vi "CRYSearch for Intersection.vi"(4 "All points":bool, 6 "Search range":string[](array[string]), 7 "Supress warnings (F)":bool, 9 "Operand B":T1={"Name"="", "Curve"=[], "X data"=1, "Y data"=1, "Z data"=1, "X axis"=0, "Y axis"=1, "Z axis"=1, "X unit"="Hz", "Y unit"="", "Z unit"="deg.", "X dB ref"=1.0, "Y dB ref"=1.0, "Z dB ref"=1.0, "single val"=FALSE, "protected"=FALSE, "display X"=TRUE, "display Y"=TRUE, "display Z"=TRUE, "Test Info"="", "Step No."=0, "Plot Settings"={"Color"=0, "Interpolation"=0, "Point Style"=0, "Line Style"=0, "Point Color"=0, "Line Width"=0, "Bar Plot Style"=0, "Fill To"=0}, "AutoProtect"=FALSE} {"Z data" items=["dB", "Lin"]; "X data" items=["dB", "Lin"]; "Y data" items=["dB", "Lin"]; "Z dB ref" format="%.1f"; "Z axis" items=["Log", "Lin"]; "X dB ref" format="%.1f"; "X axis" items=["Log", "Lin"]; "Y axis" items=["Log", "Lin"]; "Y dB ref" format="%.1f"; "Curve"."z" format="%.2f"; "Curve"."y" format="%.2f"; "Curve"."x" format="%.2f"}, 11 "Operand A":T1={"Name"="", "Curve"=[], "X data"=1, "Y data"=1, "Z data"=1, "X axis"=0, "Y axis"=1, "Z axis"=1, "X unit"="Hz", "Y unit"="", "Z unit"="deg.", "X dB ref"=1.0, "Y dB ref"=1.0, "Z dB ref"=1.0, "single val"=FALSE, "protected"=FALSE, "display X"=TRUE, "display Y"=TRUE, "display Z"=TRUE, "Test Info"="", "Step No."=0, "Plot Settings"={"Color"=0, "Interpolation"=0, "Point Style"=0, "Line Style"=0, "Point Color"=0, "Line Width"=0, "Bar Plot Style"=0, "Fill To"=0}, "AutoProtect"=FALSE} {"Z data" items=["dB", "Lin"]; "X data" items=["dB", "Lin"]; "Y data" items=["dB", "Lin"]; "Z dB ref" format="%.1f"; "Z axis" items=["Log", "Lin"]; "X dB ref" format="%.1f"; "X axis" items=["Log", "Lin"]; "Y axis" items=["Log", "Lin"]; "Y dB ref" format="%.1f"; "Curve"."z" format="%.2f"; "Curve"."y" format="%.2f"; "Curve"."x" format="%.2f"}) -> (3 "Resulting data":T1={"Name"="", "Curve"=[], "X data"=1, "Y data"=1, "Z data"=1, "X axis"=0, "Y axis"=1, "Z axis"=1, "X unit"="Hz", "Y unit"="", "Z unit"="deg.", "X dB ref"=1.0, "Y dB ref"=1.0, "Z dB ref"=1.0, "single val"=FALSE, "protected"=FALSE, "display X"=TRUE, "display Y"=TRUE, "display Z"=TRUE, "Test Info"="", "Step No."=0, "Plot Settings"={"Color"=0, "Interpolation"=0, "Point Style"=0, "Line Style"=0, "Point Color"=0, "Line Width"=0, "Bar Plot Style"=0, "Fill To"=0}, "AutoProtect"=FALSE} {"Z data" items=["dB", "Lin"]; "X data" items=["dB", "Lin"]; "Y data" items=["dB", "Lin"]; "Z dB ref" format="%.1f"; "Z axis" items=["Log", "Lin"]; "X dB ref" format="%.1f"; "X axis" items=["Log", "Lin"]; "Y axis" items=["Log", "Lin"]; "Y dB ref" format="%.1f"; "Curve"."z" format="%.2f"; "Curve"."y" format="%.2f"; "Curve"."x" format="%.2f"})   [LabVIEW 2013]
uses:
  Typedef Control/CRYData Cluster.ctl
  <vilib>/Analysis/7linalg.llb/Solve Linear Equations (single right hand).vi
  <vilib>/Analysis/baseanly.llb/Solve Linear Equations By Cholesky.vi
  <vilib>/Analysis/baseanly.llb/Real Matrix to Compact Array.vi
  <vilib>/Analysis/baseanly.llb/Real Compact Tri-Matrix Linear Eqs.vi
  <vilib>/Analysis/7linalg.llb/Solve Linear Eqs (General).vi
  <vilib>/Analysis/7linalg.llb/Solve Linear Eqs (Gen, single right hand).vi
  <vilib>/Analysis/NI_AALPro.lvlib
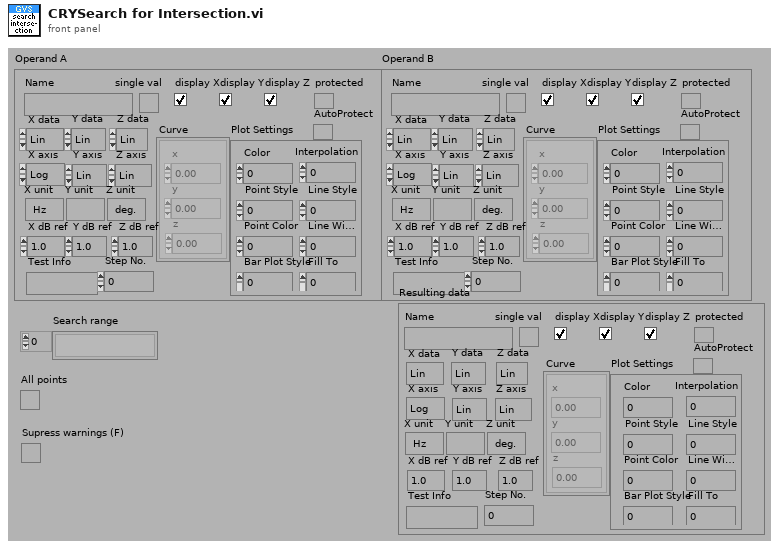
[diagram p1: front panel]
types:
  T1 = typedef "CRYData Cluster.ctl" = cluster{"Name":string, "Curve":cluster{"x":dbl, "y":dbl, "z":dbl}[], "X data":u16, "Y data":u16, "Z data":u16, "X axis":u16, "Y axis":u16, "Z axis":u16, "X unit":string, "Y unit":string, "Z unit":string, "X dB ref":dbl, "Y dB ref":dbl, "Z dB ref":dbl, "single val":bool, "protected":bool, "display X":bool, "display Y":bool, "display Z":bool, "Test Info":string, "Step No.":i32, "Plot Settings":cluster{"Color":u32, "Interpolation":u8, "Point Style":u8, "Line Style":u8, "Point Color":u32, "Line Width":u8, "Bar Plot Style":u8, "Fill To":i16}, "AutoProtect":bool}
  T2 = enum16{"OK", "Yes", "YesNo", "YesNoCancel", "ReplaceAppend"}
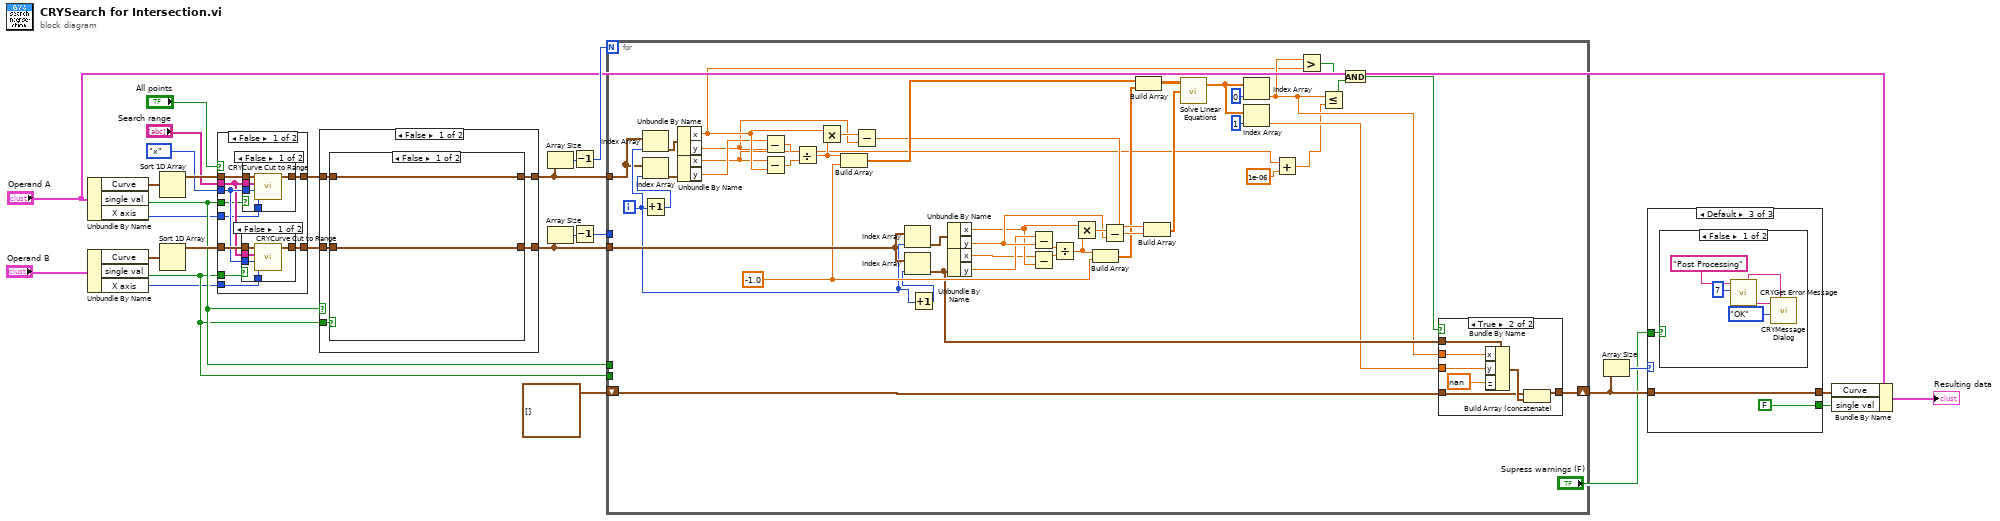
[diagram p0: block diagram]
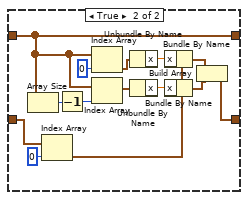
[diagram p2: hidden frame]
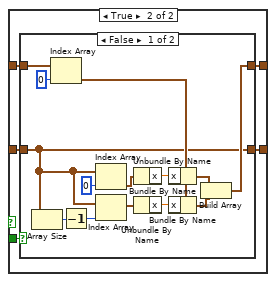
[diagram p3: hidden frame]
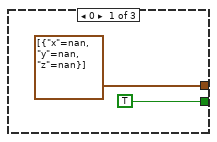
[diagram p5: hidden frame]
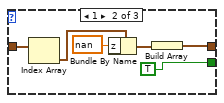
[diagram p6: hidden frame]
diagram:
  n1 = Unbundle By Name("Operand A") -> ("Curve"=w28:cluster{"x":dbl, "y":dbl, "z":dbl}[], "single val"=w9:bool, "X axis"=w7:u16)
  n2 = Unbundle By Name("Operand B") -> ("Curve"=w23:cluster{"x":dbl, "y":dbl, "z":dbl}[], "single val"=w8:bool, "X axis"=w6:u16)
  n3 = Sort 1D Array(array=w28) -> (sorted array=w27:cluster{"x":dbl, "y":dbl, "z":dbl}[])
  n4 = Sort 1D Array(array=w23) -> (sorted array=w22:cluster{"x":dbl, "y":dbl, "z":dbl}[])
  n5 = case shown="False" "All points" {
    tunnel: w27 -> [w38 w52]
    tunnel: [w37 w52] -> w13
    tunnel: enum16{"x", "y", "z"}."x" ("Range variable") -> [w35 _]
    tunnel: "Search range" -> [w34 _]
    tunnel: w22 -> [w36 w51]
    tunnel: [w33 w51] -> w11
    tunnel: w9 -> [w32 _]
    tunnel: w8 -> [w31 _]
    tunnel: w7 -> [w30 _]
    tunnel: w6 -> [w29 _]
    frame False {
      n6 = case shown="False" w31 {
        tunnel: w36 -> [w43 w44]
        tunnel: w35 -> [w42 _]
        tunnel: w34 -> [w41 _]
        tunnel: [w40 w44] -> w33
        tunnel: w29 -> [w39 _]
        frame False {
          n7 = call "CRYCurve Cut to Range.vi"("Axis type (Lin)"=w39, "Range variable (x)"=w42, "Search range"=w41, "Curve in"=w43) -> ("Cut curve out"=w40:cluster{"x":dbl, "y":dbl, "z":dbl}[])  [unwired: 7 out]
        }
        frame True {
        }
      }
      n8 = case shown="False" w32 {
        tunnel: w38 -> [w49 w50]
        tunnel: [w48 w50] -> w37
        tunnel: w35 -> [w47 _]
        tunnel: w34 -> [w46 _]
        tunnel: w30 -> [w45 _]
        frame False {
          n9 = call "CRYCurve Cut to Range.vi"("Axis type (Lin)"=w45, "Range variable (x)"=w47, "Search range"=w46, "Curve in"=w49) -> ("Cut curve out"=w48:cluster{"x":dbl, "y":dbl, "z":dbl}[])  [unwired: 7 out]
        }
        frame True {
        }
      }
    }
    frame True {
    }
  }
  n10 = case shown="False" w9 {
    tunnel: w8 -> [w57 w78]
    tunnel: w13 -> [w56 w77]
    tunnel: [w55 w76] -> w12
    tunnel: w11 -> [w54 w75]
    tunnel: [w53 w74] -> w10
    frame False {
      n11 = case shown="False" w57 {
        tunnel: [w59 w61] -> w55
        tunnel: w56 -> [w59 w61]
        tunnel: [w58 w60] -> w53
        tunnel: w54 -> [w58 w63]
        frame False {
        }
        frame True {
          n12 = Array Size(array=w61) -> (size(s)=w73:i32)
          n13 = Index Array(array=w63, index=0 ("Index")) -> (element=w62:cluster{"x":dbl, "y":dbl, "z":dbl})
          n14 = Decrement(x=w73) -> (x-1=w71:i32)
          n15 = Index Array(array=w61, index=0 ("Index")) -> (element=w69:cluster{"x":dbl, "y":dbl, "z":dbl})
          n16 = Index Array(array=w61, index=w71) -> (element=w68:cluster{"x":dbl, "y":dbl, "z":dbl})
          n17 = Unbundle By Name(w69) -> ("x"=w67:dbl)
          n18 = Unbundle By Name(w68) -> ("x"=w66:dbl)
          n19 = Bundle By Name(cluster=w62, "x"=w67) -> (w65:cluster{"x":dbl, "y":dbl, "z":dbl})
          n20 = Bundle By Name(cluster=w62, "x"=w66) -> (w64:cluster{"x":dbl, "y":dbl, "z":dbl})
          n21 = Build Array(w65, w64) -> (w60:cluster{"x":dbl, "y":dbl, "z":dbl}[])
        }
      }
    }
    frame True {
      n22 = case shown="False" w78 {
        tunnel: [w80 w94] -> w76
        tunnel: w77 -> [w88 w94]
        tunnel: [w79 w93] -> w74
        tunnel: w75 -> [w79 w93]
        frame False {
          n23 = Array Size(array=w79) -> (size(s)=w92:i32)
          n24 = Index Array(array=w88, index=0 ("Index")) -> (element=w85:cluster{"x":dbl, "y":dbl, "z":dbl})
          n25 = Decrement(x=w92) -> (x-1=w90:i32)
          n26 = Index Array(array=w79, index=0 ("Index")) -> (element=w87:cluster{"x":dbl, "y":dbl, "z":dbl})
          n27 = Index Array(array=w79, index=w90) -> (element=w86:cluster{"x":dbl, "y":dbl, "z":dbl})
          n28 = Unbundle By Name(w87) -> ("x"=w84:dbl)
          n29 = Unbundle By Name(w86) -> ("x"=w83:dbl)
          n30 = Bundle By Name(cluster=w85, "x"=w84) -> (w82:cluster{"x":dbl, "y":dbl, "z":dbl})
          n31 = Bundle By Name(cluster=w85, "x"=w83) -> (w81:cluster{"x":dbl, "y":dbl, "z":dbl})
          n32 = Build Array(w82, w81) -> (w80:cluster{"x":dbl, "y":dbl, "z":dbl}[])
        }
        frame True {
        }
      }
    }
  }
  n33 = Array Size(array=w12) -> (size(s)=w21:i32)
  n34 = Array Size(array=w10) -> (size(s)=w20:i32)
  n35 = Decrement(x=w21) -> (x-1=w19:i32)
  n36 = Decrement(x=w20) -> (x-1=w18:i32)
  n37 = for {
    N: w19 -> [_]
    tunnel: w12 -> [w108]
    tunnel: w10 -> [w136]
    tunnel: w18 -> [_]
    shift-right: [w128] -> w16
    shift-left: cluster{"x":dbl, "y":dbl, "z":dbl}[] [] -> [w127]
    tunnel: w9 -> [_]
    tunnel: w8 -> [_]
    i -> [w109]
    w130 = -1.0
    n38 = Index Array(array=w108, index=w109) -> (element=w137:cluster{"x":dbl, "y":dbl, "z":dbl})
    n39 = Increment(x=w109) -> (x+1=w138:i32)
    n40 = Index Array(array=w108, index=w138) -> (element=w107:cluster{"x":dbl, "y":dbl, "z":dbl})
    n41 = Unbundle By Name(w137) -> ("x"=w104:dbl, "y"=w98:dbl)
    n42 = Unbundle By Name(w107) -> ("x"=w96:dbl, "y"=w101:dbl)
    n43 = Subtract(x=w101, y=w98) -> (x-y=w134:dbl)
    n44 = Subtract(x=w96, y=w104) -> (x-y=w135:dbl)
    n45 = Divide(x=w134, y=w135) -> (x/y=w133:dbl)
    n46 = Multiply(x=w104, y=w133) -> (x*y=w132:dbl)
    n47 = Build Array(w133, w130) -> (w131:dbl[])
    n48 = Subtract(x=w132, y=w98) -> (x-y=w129:dbl)
    n49 = Index Array(array=w136, index=w109) -> (element=w121:cluster{"x":dbl, "y":dbl, "z":dbl})
    n50 = Increment(x=w109) -> (x+1=w126:i32)
    n51 = Index Array(array=w136, index=w126) -> (element=w106:cluster{"x":dbl, "y":dbl, "z":dbl})
    n52 = Unbundle By Name(w121) -> ("x"=w111:dbl, "y"=w113:dbl)
    n53 = Unbundle By Name(w106) -> ("x"=w110:dbl, "y"=w112:dbl)
    n54 = Subtract(x=w112, y=w113) -> (x-y=w123:dbl)
    n55 = Subtract(x=w110, y=w111) -> (x-y=w122:dbl)
    n56 = Divide(x=w123, y=w122) -> (x/y=w124:dbl)
    n57 = Multiply(x=w111, y=w124) -> (x*y=w125:dbl)
    n58 = Build Array(w124, w130) -> (w119:dbl[])
    n59 = Subtract(x=w125, y=w113) -> (x-y=w120:dbl)
    n60 = Build Array(w131, w119) -> (w118:dbl[][])
    n61 = Build Array(w129, w120) -> (w117:dbl[])
    n62 = call-poly <vilib>:"Solve Linear Equations.vi"("Known Vector"=w117, "Input Matrix"=w118) -> ("Solution Vector"=w114:dbl[])  [unwired: 1 in, 1 out]
    n63 = Index Array(array=w114, index=0 ("Index")) -> (element=w105:dbl)
    n64 = Index Array(array=w114, index=1 ("Index")) -> (element=w99:dbl)
    n65 = Add(x=w96, y=1e-06) -> (x+y=w95:dbl)
    n66 = Greater?(x=w105, y=w104) -> (0:w103:bool)
    n67 = Less Or Equal?(x=w105, y=w95) -> (x <= y?=w102:bool)
    n68 = And(x=w103, y=w102) -> (x .and. y?=w100:bool)
    n69 = case shown="True" w100 {
      tunnel: w105 -> [_ w145]
      tunnel: w99 -> [_ w144]
      tunnel: w106 -> [_ w143]
      tunnel: [w139 w141] -> w128
      tunnel: w127 -> [w139 w140]
      frame False {
      }
      frame True {
        n70 = Bundle By Name(cluster=w143, "x"=w145, "y"=w144, "z"=nan) -> (w142:cluster{"x":dbl, "y":dbl, "z":dbl})
        n71 = Build Array (concatenate)(w140, w142) -> (w141:cluster{"x":dbl, "y":dbl, "z":dbl}[])
      }
    }
  }
  n72 = Array Size(array=w16) -> (size(s)=w15:i32)
  n73 = case shown="Default" w15 {
    tunnel: w16 -> [_ w154 w155]
    tunnel: [cluster{"x":dbl, "y":dbl, "z":dbl}[] [{"x"=nan, "y"=nan, "z"=nan}] w149 w155] -> w14
    tunnel: "Supress warnings (F)" -> [_ _ w157]
    tunnel: [TRUE ("Bundle Element") TRUE ("Bundle Element") FALSE ("Bundle Element")] -> w5
    frame 0 {
    }
    frame 1 {
      n74 = Index Array(array=w154) -> (element=w153:cluster{"x":dbl, "y":dbl, "z":dbl})  [unwired: 1 in]
      n75 = Bundle By Name(cluster=w153, "z"=nan) -> (w151:cluster{"x":dbl, "y":dbl, "z":dbl})
      n76 = Build Array(w151) -> (w149:cluster{"x":dbl, "y":dbl, "z":dbl}[])
    }
    frame Default {
      n77 = case shown="False" w157 {
        frame False {
          n78 = call "CRYGet Error Message.vi"("Error No"=7, "Kind"="Post Processing") -> ("Message Sub 3"=w160:string, "Window Title"=w158:string)  [unwired: 4 in, 4 out]
          n79 = call "CRYMessage Dialog.vi"("Window Title"=w158, "YesNoCancel"=T2."OK", "Message Content"=w160) -> ()  [unwired: 7 in, 2 out]
        }
        frame True {
        }
      }
    }
  }
  n80 = Bundle By Name(cluster="Operand A", "Curve"=w14, "single val"=w5) -> (→"Resulting data":T1)
